vi "Acq Convert To Device Format.vi"(0 "session in":refnum<class "Digitizer Control.lvclass">, 1 "waveform (V)":waveform(dbl), 5 "error in (no error)":errorcluster, 6 "check for overrange? (T)":bool=TRUE, 8 "channel index":i32) -> (14 "session out":refnum<class "Digitizer Control.lvclass">, 15 "sample data":i16[](array[numeric]), 19 "error out":errorcluster)   [LabVIEW 2021, in "Digitizer Control.lvclass"]
doc: "Converts a waveform to an IQ data array of I16s that can be transferred to the FPGA Target.\n\nInputs:\n\n<B>session in</B>: The device session.\n\n<B>channel index</B>: The index of the channel whose format is to use on the <B>sample data</B> output.\n\n<B>waveform</B>: The waveform, scaled to Volts, to convert.\n\n<B>check for overrange</B>: If this input is true, then the <B>waveform</B> amplitude is checked against the amplitude range supported by the FPGA Target and an error is returned if the <B>waveform</B> amplitude is out of the supported range. The default value of this input is true.\n\nOutputs:\n\n<B>session out</B>: The device session passed on the <B>session in</B> input.\n\n<B>sample data</B>: The sample data as an array of I16s that can be transferred to the FPGA Target."
uses:
  Digitizer Control.lvclass
  Digitizer Control.lvclass/Digitizer Control.ctl
  <vilib>/Utility/error.llb/Error Cluster From Error Code.vi
  <vilib>/ErrorRing/Error Ring.xnode
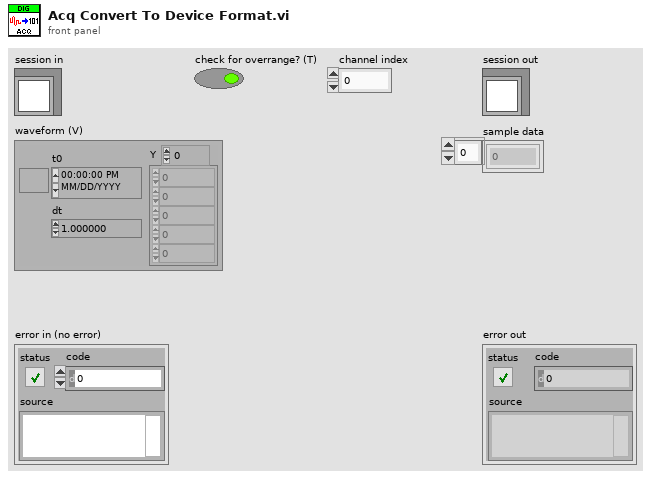
[diagram p1: front panel]
types:
  T1 = typedef "Digitizer Control.lvclass/Acq Session Data.ctl" = cluster{"ADC sampling rate":dbl, "SCTL rate":dbl, "DMA element size (bits)":i32, "sample size (bits)":i32[], "DMA/memory interface width (DMA elements)":i32, "transfer size (bits)":i32[], "stream instance":i32[], "trigger instance":u32, "group delay (s)":dbl, "data delay (s)":dbl, "target delay (s)":dbl, "trigger tracking enabled":bool, "channel configured":bool, "enabled channels":bool[], "transfer configured":bool, "dsp bypass":bool, "fractional decimator input rate":dbl, "fractional decimator output rate":dbl, "sample scale factor":dbl[], "memory size":u64[], "FIFO size":u64}
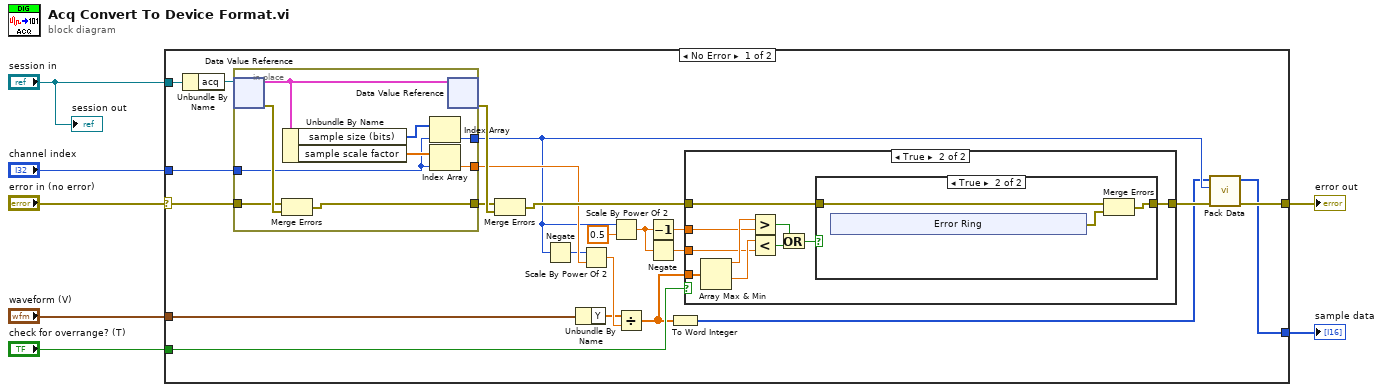
[diagram p0: block diagram]
diagram:
  n1 = case shown="No Error" "error in (no error)" {
    selector: "error in (no error)" -> [w23 w60]
    tunnel: [w28 w60] -> w6
    tunnel: "waveform (V)" -> [w26 _]
    tunnel: "check for overrange? (T)" -> [w25 _]
    tunnel: "session in" -> [w21 _]
    tunnel: [w14 _] -> w2
    tunnel: "channel index" -> [w13 _]
    frame No Error {
      n2 = Unbundle By Name(w21) -> ("acq"=w20:refnum<data-value>)
      n3 = in-place {
        in-place-border: w23 -> [w38]
        in-place-border: [w37] -> w22
        in-place-border: [w34] -> w17
        in-place-border: [w31] -> w12
        in-place-border: w13 -> [w33]
        n4 = in-place-dvr #1(w20) -> (w36:T1, w39:errorcluster)
        n5 = Merge Errors(w38, w39) -> (w37:errorcluster)
        n6 = Unbundle By Name(w36) -> ("sample size (bits)"=w32:i32[], "sample scale factor"=w35:dbl[])
        n7 = Index Array(array=w32, index=w33) -> (element=w31:i32)
        n8 = Index Array(array=w35, index=w33) -> (element=w34:dbl)
        n9 = in-place-dvr #1(w36) -> (w27:errorcluster)  [unwired: 1 out]
      }
      n10 = Merge Errors(w22, w27) -> (w30:errorcluster)
      n11 = Negate(x=w12) -> (-x=w16:i32)
      n12 = Unbundle By Name(w26) -> ("Y"=w11:dbl[])
      n13 = Scale By Power Of 2(n=w16, x=w17) -> (x*2^n=w15:dbl)
      n14 = Scale By Power Of 2(n=w12, x=0.5) -> (x*2^n=w9:dbl)
      n15 = Divide(x=w11, y=w15) -> (x/y=w24:dbl[])
      n16 = Decrement(x=w9) -> (x-1=w18:dbl)
      n17 = Negate(x=w9) -> (-x=w8:dbl)
      n18 = To Word Integer(number=w24) -> (16bit integer=w10:i16[])
      n19 = case shown="True" w25 {
        tunnel: w24 -> [_ w46]
        tunnel: w30 -> [w40 w49]
        tunnel: [w40 w48] -> w29
        tunnel: w18 -> [_ w47]
        tunnel: w8 -> [_ w44]
        frame False {
        }
        frame True {
          n20 = Array Max & Min(array=w46) -> (max value=w50:dbl, min value=w45:dbl)  [unwired: 2 out]
          n21 = Greater?(x=w50, y=w47) -> (0:w42:bool)
          n22 = Less?(x=w45, y=w44) -> (x < y?=w43:bool)
          n23 = Or(x=w42, y=w43) -> (x .or. y?=w41:bool)
          n24 = case shown="True" w41 {
            tunnel: w49 -> [w51 w54]
            tunnel: [w51 w52] -> w48
            frame False {
            }
            frame True {
              n25 = xnode "Error Ring"() -> ("error out"=w53:errorcluster)
              n26 = Merge Errors(w54, w53) -> (w52:errorcluster)
            }
          }
        }
      }
      n27 = call "Pack Data.vi"("error in (no error)"=w29, "packed data size (bits)"=w12, "unpacked data in"=w10) -> ("error out"=w28:errorcluster, "packed data out"=w14:i16[])  [unwired: 7 in]
    }
    frame Error {
    }
  }
  "error out" <- w6
  "sample data" <- w2
  "session out" <- "session in"
